vi "手柄控制.vi"() -> ()   [LabVIEW 2016]
uses:
  <vilib>/Utility/inputDevices.llb/joystickAcquire.vi
  <vilib>/Utility/inputDevices.llb/closeJoystick.vi
panel:
  out "axis info":T1 caption="坐标轴信息"
  out "direction info":T2 caption="方向信息"
  out "button info":T3 caption="按钮信息"
  in  "停止按钮":bool
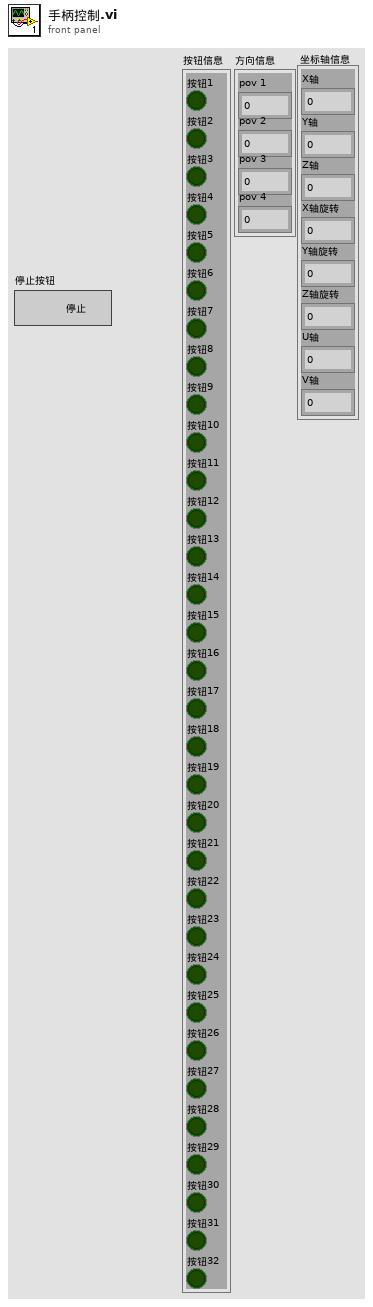
[diagram p1: front panel]
types:
  T1 = cluster{"X axis":i32, "Y axis":i32, "Z axis":i32, "X axis rotation":i32, "Y axis rotation":i32, "Z axis rotation":i32, "U axis":i32, "V axis":i32}
  T2 = cluster{"pov 1":i32, "pov 2":i32, "pov 3":i32, "pov 4":i32}
  T3 = cluster{"button 1":bool, "button 2":bool, "button 3":bool, "button 4":bool, "button 5":bool, "button 6":bool, "button 7":bool, "button 8":bool, "button 9":bool, "button 10":bool, "button 11":bool, "button 12":bool, "button 13":bool, "button 14":bool, "button 15":bool, "button 16":bool, "button 17":bool, "button 18":bool, "button 19":bool, "button 20":bool, "button 21":bool, "button 22":bool, "button 23":bool, "button 24":bool, "button 25":bool, "button 26":bool, "button 27":bool, "button 28":bool, "button 29":bool, "button 30":bool, "button 31":bool, "button 32":bool}
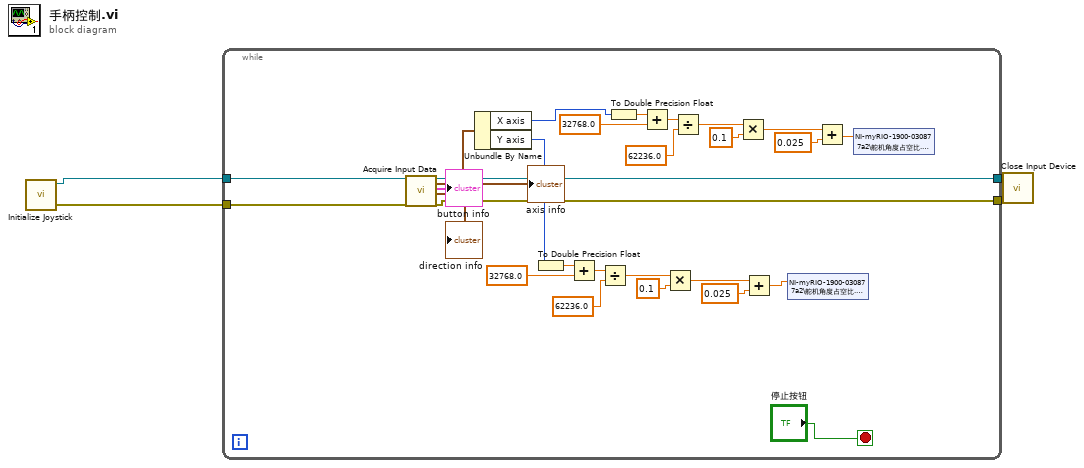
[diagram p0: block diagram]
diagram:
  n1 = call <vilib>:"Initialize Joystick.vi"() -> ("error out"=w3:errorcluster, "device ID"=w4:refnum<k1>)  [unwired: 10 in]
  n2 = while {
    tunnel: w4 -> [w32]
    tunnel: w3 -> [w31]
    tunnel: [w30] -> w2
    tunnel: [w29] -> w1
    stop <- "停止按钮" stop-if-true
    n3 = call-poly <vilib>:"Acquire Input Data.vi"("device ID"=w32, "error in (no error)"=w31) -> ("device ID"=w30:refnum<k1>, "axis info"=w27:T1, "button info"=→"button info":T3, "direction info"=→"direction info":T2, "error out"=w29:errorcluster)  [unwired: 13 in]
    "axis info" <- w27
    n4 = Unbundle By Name(w27) -> ("X axis"=w25:i32, "Y axis"=w17:i32)
    n5 = To Double Precision Float(number=w17) -> (double precision float=w15:dbl)
    n6 = Add(x=w15, y=32768.0) -> (x+y=w14:dbl)
    n7 = Divide(x=w14, y=62236.0) -> (x/y=w12:dbl)
    n8 = To Double Precision Float(number=w25) -> (double precision float=w24:dbl)
    n9 = Add(x=w24, y=32768.0) -> (x+y=w26:dbl)
    n10 = Multiply(x=w12, y=0.1) -> (x*y=w10:dbl)
    n11 = Divide(x=w26, y=62236.0) -> (x/y=w21:dbl)
    n12 = Multiply(x=w21, y=0.1) -> (x*y=w19:dbl)
    n13 = Add(x=w10, y=0.025) -> (x+y=w8:dbl)
    n14 = shared-variable "NI-myRIO-1900-030877a2\\舵机角度占空比.lvlib\\上舵机"(w8) -> ()  [unwired: 1 in, 1 out]
    n15 = Add(x=w19, y=0.025) -> (x+y=w7:dbl)
    n16 = shared-variable "NI-myRIO-1900-030877a2\\舵机角度占空比.lvlib\\下舵机"(w7) -> ()  [unwired: 1 in, 1 out]
  }
  n17 = call-poly <vilib>:"Close Input Device.vi"("error in (no error)"=w1, "device ID"=w2) -> ()  [unwired: 8 in, 1 out]
